vi "CSVQuoteField.vi"(8 "error in (no error)":errorcluster, 10 "delimiter":string, 11 "field":string) -> (0 "error out":errorcluster, 3 "quotedField":string)   [LabVIEW 2026, in "Lumberjack.lvlib"]
uses:
  Lumberjack.lvlib
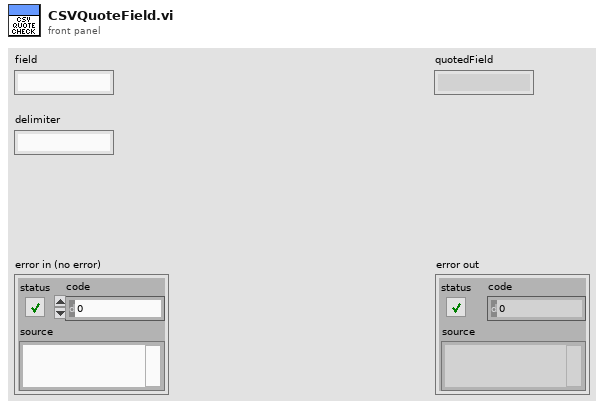
[diagram p1: front panel]
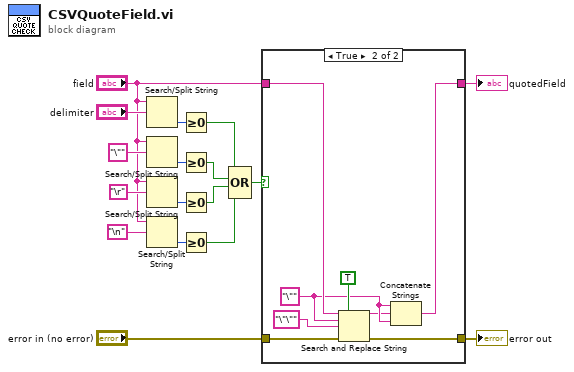
[diagram p0: block diagram]
diagram:
  n1 = Search/Split String(string="field", search string/char (-)="delimiter") -> (offset of match=w13:i32)  [unwired: 1 in, 2 out]
  n2 = Search/Split String(string="field", search string/char (-)="\"") -> (offset of match=w12:i32)  [unwired: 1 in, 2 out]
  n3 = Search/Split String(string="field", search string/char (-)="\r") -> (offset of match=w11:i32)  [unwired: 1 in, 2 out]
  n4 = Search/Split String(string="field", search string/char (-)="\n") -> (offset of match=w10:i32)  [unwired: 1 in, 2 out]
  n5 = Greater Or Equal To 0?(x=w13) -> (x >= 0?=w5:bool)
  n6 = Greater Or Equal To 0?(x=w12) -> (x >= 0?=w3:bool)
  n7 = Greater Or Equal To 0?(x=w11) -> (x >= 0?=w2:bool)
  n8 = Greater Or Equal To 0?(x=w10) -> (x >= 0?=w4:bool)
  n9 = Compound Arithmetic op=OR(w5, w3, w2, w4) -> (w1:bool)
  n10 = case shown="True" w1 {
    tunnel: "error in (no error)" -> [w18 w27]
    tunnel: [w18 w26] -> w8
    tunnel: [w19 w20] -> w7
    tunnel: "field" -> [w19 w25]
    frame False {
    }
    frame True {
      w22 = "\"" ("search string")
      n11 = Search and Replace String(replace all?=TRUE ("replace all? (F)"), input string=w25, search string=w22, replace string="\"\"" ("replace string (\"\")"), error in=w27) -> (result string=w21:string, error out=w26:errorcluster)  [unwired: 3 in, 2 out]
      n12 = Concatenate Strings(w22, w21, w22) -> (w20:string)
    }
  }
  "quotedField" <- w7
  "error out" <- w8
